vi "CubeLiftInit.vi"   [LabVIEW 2017]
uses:
  <vilib>/Rock Robotics/WPI/Solenoid/WPI_SolenoidChannel.ctl
  <vilib>/Rock Robotics/WPI/ThirdParty/Phoenix-LabVIEW/Motor Controller/Controls/CTRE_Phoenix_MotorControl_StatusFrameEnhanced.ctl
  <vilib>/Rock Robotics/WPI/ThirdParty/Phoenix-LabVIEW/Motor Controller/Controls/CTRE_Phoenix_MotorControl_FeedbackDevice.ctl
  <vilib>/Rock Robotics/WPI/ThirdParty/Phoenix-LabVIEW/Motor Controller/Controls/CTRE_Phoenix_MotorControl_NeutralMode.ctl
  CubeLiftCommand.ctl
  RunMode.ctl
  <vilib>/Rock Robotics/WPI/Solenoid/WPI_SolenoidValue.ctl
  <vilib>/Rock Robotics/WPI/Solenoid/WPI_SolenoidOpenSingle.vi
  <vilib>/Rock Robotics/WPI/Solenoid/WPI_SolenoidSetEnum.vi
  Robot Global Data.vi
types:
  T1 = typedef "WPI_SolenoidChannel.ctl" = enum8{"Solenoid 0", "Solenoid 1", "Solenoid 2", "Solenoid 3", "Solenoid 4", "Solenoid 5", "Solenoid 6", "Solenoid 7", "Invalid"}
  T2 = typedef "WPI_SolenoidValue.ctl" = enum16{"Off", "On", "Forward", "Reverse"}
  T3 = typedef "CubeLiftCommand.ctl" = cluster{"Bucket":cluster{"Deposit":bool}, "Slide":cluster{"Slide command":enum16{"Up", "Down", "Stationary"}}, "Mode":T4}
  T4 = typedef "RunMode.ctl" = enum16{"Auto", "Teleop", "Disabled"}
  T5 = typedef "CTRE_Phoenix_MotorControl_NeutralMode.ctl" = enum8{"EEPROMSetting", "Override to Coast", "Override to Brake"}
  T6 = typedef "CTRE_Phoenix_MotorControl_FeedbackDevice.ctl" = i8
  T7 = typedef "CTRE_Phoenix_MotorControl_StatusFrameEnhanced.ctl" = u16
  T8 = typedef "WPI_MotorControlDeviceRef.ctl" = cluster{"DeviceStatus":errorcluster, "Type":T9, "PWM":cluster{"PWM Channel":T10, "DeadBand":T11}, "CAN":cluster{"Device Number":u8, "SetOutput VI Ref":variant, "GetOutput VI Ref":variant, "Enable VI Ref":variant, "Disable VI Ref":variant, "Data":variant}, "Invert":bool, "DIO PWM":cluster{"PWM \"Enable\" Channel":T10, "DIOChannel":T12, "PWM Rate":dbl}}
  T9 = typedef "WPI_MotorControlType.ctl" = enum16{"PWM", "CAN", "DIO PWM"}
  T10 = typedef "FPGA_DIOPWMChannel.ctl" = enum8{"PWM 0", "PWM 1", "PWM 2", "PWM 3", "PWM 4", "PWM 5", "PWM 6", "PWM 7", "PWM 8", "PWM 9", "PWM MXP 0", "PWM MXP 1", "PWM MXP 2", "PWM MXP 3", "PWM MXP 4", "PWM MXP 5", "PWM MXP 6", "PWM MXP 7", "PWM MXP 8", "PWM MXP 9", "Invalid"}
  T11 = typedef "WPI_PWMDeadband.ctl" = cluster{"Name":string, "maxPositivePwm":i32, "minPositivePwm":i32, "centerPwm":i32, "maxNegativePwm":i32, "minNegativePwm":i32, "angularRange":u16}
  T12 = typedef "FPGA_DIOChannel.ctl" = enum8{"DIO 0", "DIO 1", "DIO 2", "DIO 3", "DIO 4", "DIO 5", "DIO 6", "DIO 7", "DIO 8", "DIO 9", "DIO MXP 0", "DIO MXP 1", "DIO MXP 2", "DIO MXP 3", "DIO MXP 4", "DIO MXP 5", "DIO MXP 6", "DIO MXP 7", "DIO MXP 8", "DIO MXP 9", "DIO MXP 10", "DIO MXP 11", "DIO MXP 12", "DIO MXP 13", "DIO MXP 14", "DIO MXP 15", "SPI Port CS1", "SPI Port CS2", "SPI Port CS3", "SPI Port MISO", "SPI Port MOSI", "Invalid"}
  T13 = typedef "WPI_SolenoidDevRef.ctl" = cluster{"DevStatus":errorcluster, "Pneumatics Control Module":u8, "Forward Solenoid Channel":T1, "Reverse Solenoid Channel":T1}
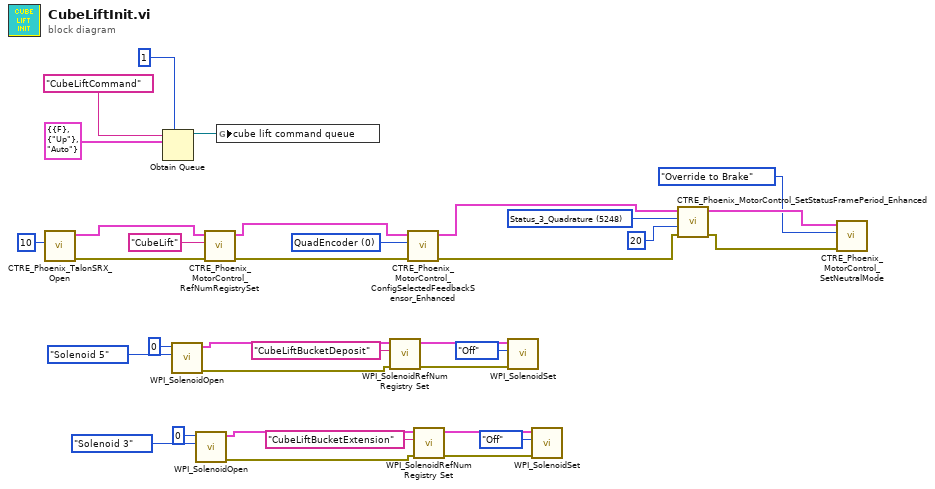
[diagram p0: block diagram]
diagram:
  w20 = T6 0 items=["None"=-1, "QuadEncoder"=0, "Analog"=2, "Tachometer"=4, "Pulse Width Encoded Position"=8, "Sensor Sum (S0 + S1)"=9, "Sensor Difference (D0 - D1)"=10, "Remote Source 0"=11, "Remote Source 1"=12, "Software Emulated"=15] ("Feedback Device")
  w23 = T7 5248 items=["Status_1_General"=5120, "Status_2_Feedback0"=5184, "Status_3_Quadrature"=5248, "Status_4_AinTempVbat"=5312, "Status_6_Misc"=5440, "Status_7_CommStatus"=5504, "Status_8_PulseWidth"=5568, "Status_9_MotProfBuffer"=5632, "Status_10_MotionMagic"=5696, "Status_11_UartGadgeteer"=5760, "Status_12_Feedback1"=5824, "Status_13_Base_PIDF0"=5888, "Status_14_Turn_PIDF1"=5952, "Status_15_FirmwareApiStatus"=6016] ("Status Frame")
  n1 = call <vilib>:"CTRE_Phoenix_TalonSRX_Open.vi"("Device Number"=u8 10) -> ("error out"=w21:errorcluster, "CAN Talon SRX Ref"=w33:T8)  [unwired: 9 in]
  n2 = Obtain Queue(max queue size (-1, unlimited)=1, name (unnamed)="CubeLiftCommand", element data type=T3 {"Bucket"={"Deposit"=FALSE}, "Slide"={"Slide command"=enum."Up"}, "Mode"=enum."Auto"} ("Cube Lift Command")) -> (queue out=w9:refnum<queue>)  [unwired: 2 in, 2 out]
  n3 = call-poly <vilib>:"WPI_SolenoidOpen.vi"("Solenoid Channel"=WPI_SolenoidChannel."Solenoid 5", "Pneumatics Control Module (0)"=u8 0) -> ("error out"=w27:errorcluster, "SolenoidDevRef"=w26:T13)  [unwired: 8 in]
  n4 = call-poly <vilib>:"WPI_SolenoidOpen.vi"("Solenoid Channel"=WPI_SolenoidChannel."Solenoid 3", "Pneumatics Control Module (0)"=u8 0) -> ("error out"=w4:errorcluster, "SolenoidDevRef"=w3:T13)  [unwired: 8 in]
  n5 = call <vilib>:"CTRE_Phoenix_MotorControl_RefNumRegistrySet.vi"("error in (no error)"=w21, "refnum name"="CubeLift", "PhoenixMotorControlDevRef"=w33) -> ("error out"=w18:errorcluster, "PhoenixMotorControlDevRef"=w19:T8)  [unwired: 7 in]
  n6 = global write "Robot Global Data.vi" "cube lift command queue"(w9) -> ()
  n7 = call <vilib>:"WPI_SolenoidRefNum Registry Set.vi"("error in (no error)"=w27, "refnum name"="CubeLiftBucketDeposit", "SolenoidDevRef"=w26) -> ("error out"=w31:errorcluster, "SolenoidDevRef"=w30:T13)  [unwired: 7 in]
  n8 = call <vilib>:"CTRE_Phoenix_MotorControl_ConfigSelectedFeedbackSensor_Enhanced.vi"("error in (no error)"=w18, "Feedback Device"=w20, "PhoenixMotorControlDevRef"=w19) -> ("error out"=w17:errorcluster, "PhoenixMotorControlDevRef"=w16:T8)  [unwired: 7 in]
  n9 = call <vilib>:"WPI_SolenoidRefNum Registry Set.vi"("error in (no error)"=w4, "refnum name"="CubeLiftBucketExtension", "SolenoidDevRef"=w3) -> ("error out"=w8:errorcluster, "SolenoidDevRef"=w7:T13)  [unwired: 7 in]
  n10 = call-poly <vilib>:"WPI_SolenoidSet.vi"("error in (no error)"=w31, "Value"=WPI_SolenoidValue."Off", "SolenoidDevRef"=w30) -> ()  [unwired: 7 in, 2 out]
  n11 = call-poly <vilib>:"WPI_SolenoidSet.vi"("error in (no error)"=w8, "Value"=WPI_SolenoidValue."Off", "SolenoidDevRef"=w7) -> ()  [unwired: 7 in, 2 out]
  n12 = call <vilib>:"CTRE_Phoenix_MotorControl_SetStatusFramePeriod_Enhanced.vi"("error in (no error)"=w17, "periodMs"=20, "Status Frame"=w23, "PhoenixMotorControlDevRef"=w16) -> ("error out"=w14:errorcluster, "PhoenixMotorControlDevRef"=w15:T8)  [unwired: 6 in]
  n13 = call <vilib>:"CTRE_Phoenix_MotorControl_SetNeutralMode.vi"("error in (no error)"=w14, "Motor Control Neutral Mode"=CTRE_Phoenix_MotorControl_NeutralMode."Override to Brake", "PhoenixMotorControlDevRef"=w15) -> ()  [unwired: 7 in, 2 out]
